vi "Load Single Level.vi"(8 "error in (no error)":errorcluster, 10 "Tag":string, 11 "TreeDirectory in":refnum<class "TreeDirectory.lvclass">) -> (0 "error out":errorcluster, 3 "Tree (dup)":refnum<class "TreeDirectory.lvclass">)   [LabVIEW 2015, in "TreeDirectory.lvclass"]
uses:
  TreeDirectory.lvclass
  TreeControl/Add Item Info Cluster.ctl
  TreeDirectory.lvclass/TreeDirectory.ctl
  TreeControl/Tree Action Enum.ctl
  TreeControl/TreeControl.lvclass
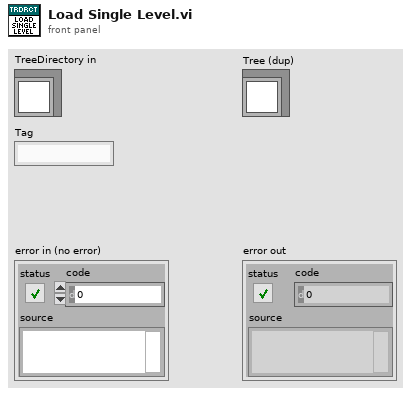
[diagram p1: front panel]
types:
  T1 = typedef "TreeControl.lvclass/Add Item Info Cluster.ctl" = cluster{"Parent Tag (\"\")":string, "Child Position (-1=End)":i32, "Left Cell String (\"\" = Same as Child Tag)":string, "Child Text[]":string[], "Child Tag":string, "Child Only? (F)":bool}
  T2 = typedef "TreeControl.lvclass/Tree Action Enum.ctl" = enum16{"Open All", "Close All", "Open Item", "Close Item"}
  T3 = typedef "imagedata.ctl" = cluster{"image type":i32, "image depth":i32, "image":u8[], "mask":u8[], "colors":u32[], "Rectangle":cluster{"left":i16, "top":i16, "right":i16, "bottom":i16}}
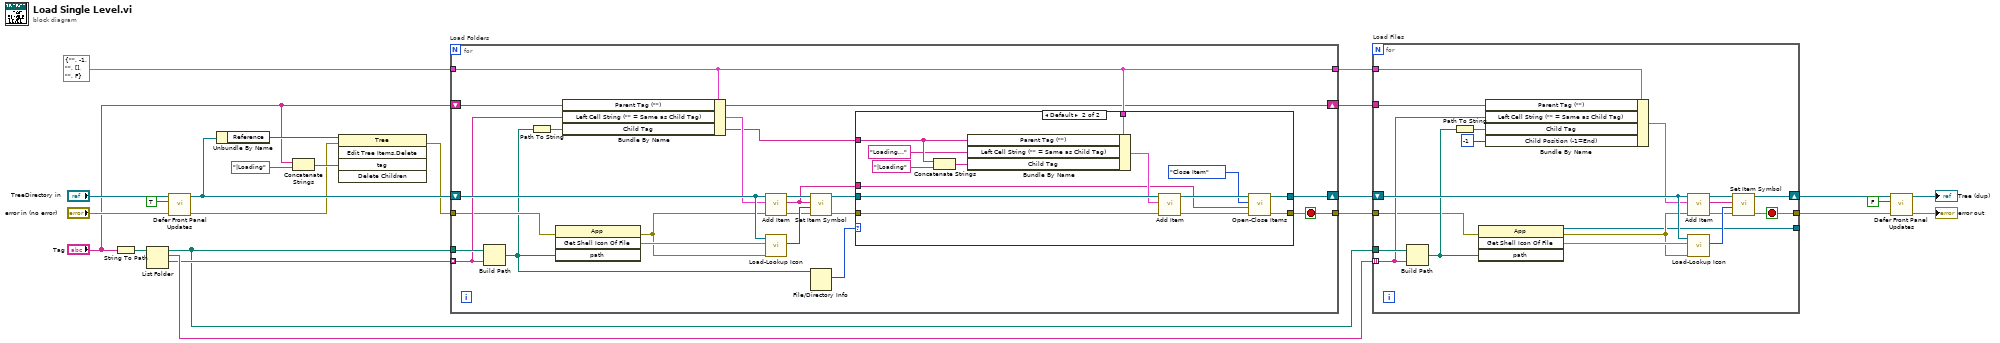
[diagram p0: block diagram]
diagram:
  n1 = String To Path(string="Tag") -> (path=w6:path)
  n2 = List Folder(path=w6) -> (path out=w18:path, filenames=w24:string[], folder names=w23:string[])  [unwired: 3 in, 1 out]
  n3 = call "Defer Front Panel Updates.vi"("error in (no error)"="error in (no error)", "Defer Panel Updates (F)"=TRUE, "Tree in"="TreeDirectory in") -> ("error out"=w9:errorcluster, "Tree (dup)"=w13:refnum<class "TreeDirectory.lvclass">)  [unwired: 7 in]
  n4 = Unbundle By Name(w13) -> ("Reference"=w12:refnum<vi>)
  n5 = Concatenate Strings("Tag", "|Loading" ("string")) -> (w10:string)
  n6 = invoke class="Tree" method="Edit Tree Items.Delete"(reference=w12, error in=w9, "tag"=w10) -> (error out=w8:errorcluster)  [unwired: 2 in, 4 out]
  n7 = for "Load Folders" {
    tunnel: w23 -> [w40] mode=indexing
    shift-right: [w32] -> w22
    shift-left: w13 -> [w42]
    tunnel: w18 -> [w44]
    tunnel: T1 {"Parent Tag (\"\")"="", "Child Position (-1=End)"=-1, "Left Cell String (\"\" = Same as Child Tag)"="", "Child Text[]"=[], "Child Tag"="", "Child Only? (F)"=FALSE} ("ItemInfo") -> [w34]
    tunnel: [w34] -> w20
    tunnel: [w31] -> w2
    tunnel: w8 -> [w30]
    shift-right: [w27] -> w19
    shift-left: "Tag" -> [w27]
    stop <- w31 stop-if-true
    n8 = Build Path(base path=w44, name or relative path=w40) -> (appended path=w26:path)
    n9 = Path To String(path=w26) -> (string=w38:string)
    n10 = invoke class="App" method="Get Shell Icon Of File"(error in=w30, "path"=w26) -> (error out=w28:errorcluster, "GetShellIconOfFile"=w29:T3)  [unwired: 2 in, 2 out]
    n11 = Bundle By Name(cluster=w34, "Parent Tag (\"\")"=w27, "Left Cell String (\"\" = Same as Child Tag)"=w40, "Child Tag"=w38) -> (w39:T1)
    n12 = call-dynamic "Add Item.vi"("error in (no error)"=w28, "ItemInfo"=w39, "Tree in"=w42) -> ("error out"=w35:errorcluster, "Add Item Tag"=w33:string, "Tree (dup)"=w41:refnum<class "TreeDirectory.lvclass">)  [unwired: 6 in]
    n13 = call "Load-Lookup Icon.vi"("error in (no error)"=w28, "Shell Icon"=w29, "TreeDirectory in"=w42) -> ("Icon Index"=w43:i32)  [unwired: 6 in, 2 out]
    n14 = call "Set Item Symbol.vi"("error in (no error)"=w35, "Symbol Index"=w43, "Tag"=w33, "Tree in"=w41) -> ("error out"=w36:errorcluster, "Tree (dup)"=w37:refnum<class "TreeDirectory.lvclass">)  [unwired: 6 in]
    n15 = File/Directory Info(path=w26) -> (size=w25:i64)  [unwired: 1 in, 6 out]
    n16 = case shown="Default" w25 {
      tunnel: w38 -> [_ w60]
      tunnel: w37 -> [w46 w56]
      tunnel: w36 -> [w45 w54]
      tunnel: w34 -> [_ w53]
      tunnel: w33 -> [_ w50]
      tunnel: [w46 w48] -> w32
      tunnel: [w45 w47] -> w31
      frame 0 {
      }
      frame Default {
        n17 = Concatenate Strings(w60, "|Loading" ("string")) -> (w58:string)
        n18 = Bundle By Name(cluster=w53, "Parent Tag (\"\")"=w60, "Left Cell String (\"\" = Same as Child Tag)"="Loading..." ("string"), "Child Tag"=w58) -> (w55:T1)
        n19 = call-dynamic "Add Item.vi"("error in (no error)"=w54, "ItemInfo"=w55, "Tree in"=w56) -> ("error out"=w49:errorcluster, "Tree (dup)"=w52:refnum<class "TreeDirectory.lvclass">)  [unwired: 6 in, 1 out]
        n20 = call-dynamic "Open-Close Items.vi"("error in (no error)"=w49, "Tag (\"\")"=w50, "Action (Close All)"=Tree_Action_Enum."Close Item", "Tree in"=w52) -> ("error out"=w47:errorcluster, "Tree (dup)"=w48:refnum<class "TreeDirectory.lvclass">)  [unwired: 6 in]
      }
    }
  }
  n21 = for "Load Files" {
    tunnel: w24 -> [w73] mode=indexing
    shift-right: [w66] -> w14
    shift-left: w22 -> [w76]
    tunnel: w18 -> [w79]
    tunnel: w20 -> [w70]
    tunnel: w19 -> [w67]
    tunnel: w2 -> [w65]
    tunnel: [w63] -> w3
    tunnel: [w62] -> _
    stop <- w63 stop-if-true
    n22 = Build Path(base path=w79, name or relative path=w73) -> (appended path=w72:path)
    n23 = Path To String(path=w72) -> (string=w69:string)
    n24 = invoke class="App" method="Get Shell Icon Of File"(error in=w65, "path"=w72) -> (reference out=w62:refnum<vi>, error out=w64:errorcluster, "GetShellIconOfFile"=w78:T3)  [unwired: 2 in, 1 out]
    n25 = Bundle By Name(cluster=w70, "Parent Tag (\"\")"=w67, "Left Cell String (\"\" = Same as Child Tag)"=w73, "Child Tag"=w69, "Child Position (-1=End)"=-1) -> (w71:T1)
    n26 = call-dynamic "Add Item.vi"("error in (no error)"=w64, "ItemInfo"=w71, "Tree in"=w76) -> ("error out"=w68:errorcluster, "Add Item Tag"=w74:string, "Tree (dup)"=w75:refnum<class "TreeDirectory.lvclass">)  [unwired: 6 in]
    n27 = call "Load-Lookup Icon.vi"("error in (no error)"=w64, "Shell Icon"=w78, "TreeDirectory in"=w76) -> ("Icon Index"=w77:i32)  [unwired: 6 in, 2 out]
    n28 = call "Set Item Symbol.vi"("error in (no error)"=w68, "Symbol Index"=w77, "Tag"=w74, "Tree in"=w75) -> ("error out"=w63:errorcluster, "Tree (dup)"=w66:refnum<class "TreeDirectory.lvclass">)  [unwired: 6 in]
  }
  n29 = call "Defer Front Panel Updates.vi"("error in (no error)"=w3, "Defer Panel Updates (F)"=FALSE, "Tree in"=w14) -> ("error out"=→"error out":errorcluster, "Tree (dup)"=→"Tree (dup)":refnum<class "TreeDirectory.lvclass">)  [unwired: 7 in]
